vi "RoundLED_0222.vi"() -> ()   [LabVIEW 2018]
panel:
  out "Waveform Chart":dbl(graph)
  out "error out":errorcluster
  in  "error in (no error)":errorcluster
  out "Boolean":bool
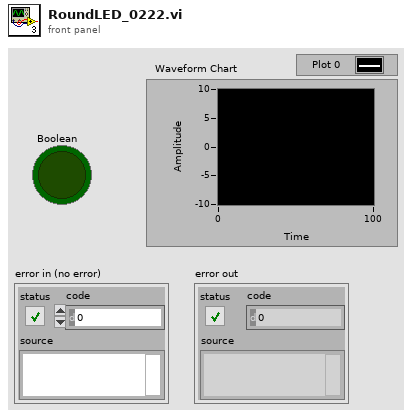
[diagram p1: front panel]
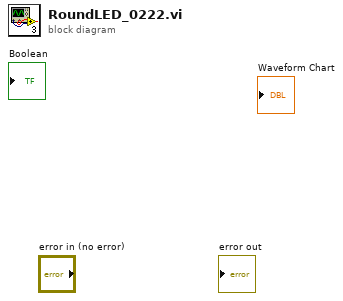
[diagram p0: block diagram]
diagram:
